vi "Get Model Number.vi"(11 "Barcode":string) -> (2 "Found?":bool, 3 "Model Number":string)   [LabVIEW 2021, in "Sequence Engine.lvlib"]
uses:
  Sequence Engine.lvlib
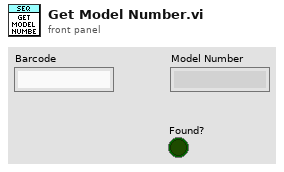
[diagram p1: front panel]
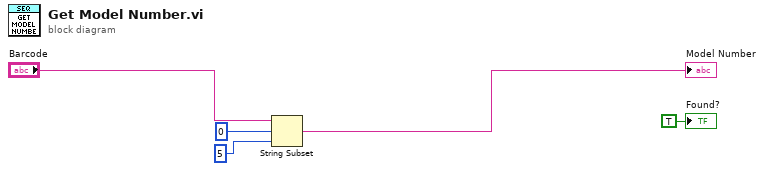
[diagram p0: block diagram]
diagram:
  n1 = String Subset(string="Barcode", offset (0)=0, length (rest)=5 ("length (rest)")) -> (substring=→"Model Number":string)
  "Found?" <- TRUE ("Found?")
